vi "Tail Follow.vi"(7 "Head":T1, 11 "Tail":T1) -> (3 "Tail Out":T1)   [LabVIEW 2020]
uses:
  Cluster_Point.ctl
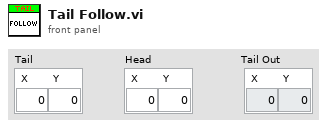
[diagram p1: front panel]
types:
  T1 = typedef "Cluster_Point.ctl" = cluster{"X":i32, "Y":i32}
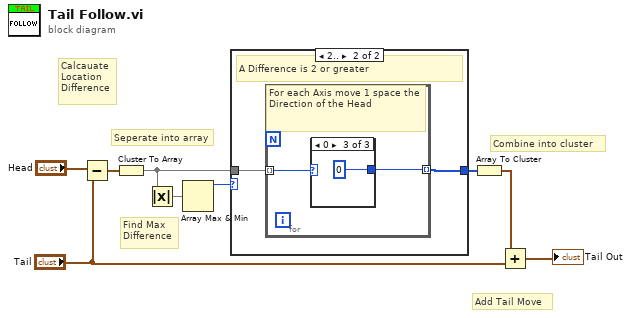
[diagram p0: block diagram]
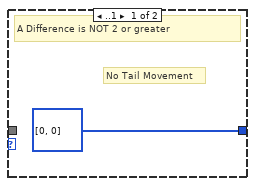
[diagram p2: hidden frame]
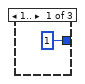
[diagram p3: hidden frame]
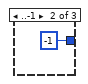
[diagram p4: hidden frame]
diagram:
  # "Add Tail Move"
  # "Find Max\nDifference"
  # "Combine into cluster"
  # "Seperate into array"
  # "Calcauate\nLocation\nDifference"
  n1 = Subtract(x="Head", y="Tail") -> (x-y=w4:T1)
  n2 = Cluster To Array(cluster=w4) -> (array=w3:i32[])
  n3 = Absolute Value(x=w3) -> (abs(x)=w2:i32[])
  n4 = Array Max & Min(array=w2) -> (max value=w1:i32)  [unwired: 3 out]
  n5 = case shown="2.." w1 {
    tunnel: [i32[] [0, 0] w12] -> w8
    tunnel: w3 -> [_ w11]
    frame ..1 {
      # "No Tail Movement"
      # "A Difference is NOT 2 or greater"
    }
    frame 2.. {
      # "A Difference is 2 or greater"
      n6 = for {
        tunnel: w11 -> [w14] mode=indexing
        tunnel: [w13] -> w12 mode=indexing
        # "For each Axis move 1 space the Direction of the Head"
        n7 = case shown="0" w14 {
          tunnel: [1 -1 0] -> w13
          frame 1.. {
          }
          frame ..-1 {
          }
          frame 0 {
          }
        }
      }
    }
  }
  n8 = Array To Cluster(array=w8) -> (cluster=w7:cluster{"[0]":i32, "[1]":i32})
  n9 = Add(x=w7, y="Tail") -> (x+y=→"Tail Out":T1)
